vi "Bcalc.vi"(1 "baseR":dbl=0.088) -> (0 "B":T1)   [LabVIEW 2019]
uses:
  <vilib>/Analysis/Matrix/Datatypes/RealMatrix.ctl
  <vilib>/Analysis/Matrix/NI_Matrix.lvlib
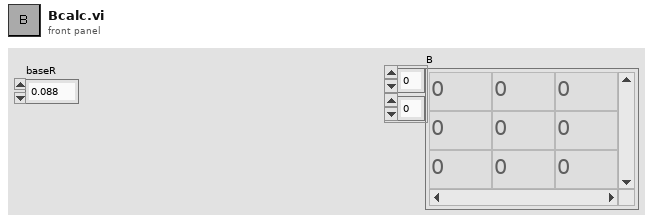
[diagram p1: front panel]
types:
  T1 = typedef "NI_Matrix.lvlib/RealMatrix.ctl" = dbl[][]
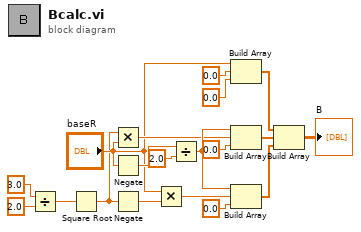
[diagram p0: block diagram]
diagram:
  n1 = Divide(x=3.0, y=2.0) -> (x/y=w11:dbl)
  n2 = Square Root(x=w11) -> (sqrt(x)=w4:dbl)
  n3 = Multiply(x=w4, y="baseR") -> (x*y=w6:dbl)
  n4 = Negate(x="baseR") -> (-x=w15:dbl)
  n5 = Negate(x=w4) -> (-x=w10:dbl)
  n6 = Multiply(x="baseR", y=w10) -> (x*y=w9:dbl)
  n7 = Divide(x=w15, y=2.0) -> (x/y=w7:dbl)
  n8 = Build Array("baseR", 0.0, 0.0) -> (w17:dbl[])
  n9 = Build Array(w7, w6, 0.0 ("element")) -> (w3:dbl[])
  n10 = Build Array(w7, w9, 0.0 ("element")) -> (w2:dbl[])
  n11 = Build Array(w17, w3, w2) -> (→"B":T1)
